vi "Example_CustomCursors.vi"() -> ()   [LabVIEW 2020, in "LcPictureBox.lvclass"]
uses:
  LcPictureBox.lvclass
  SmoothingMode.ctl
  Pen.ctl
  ce328d88-1fef-4cb5-b4df-921596365a82.vi
  1ca8d7fc-782b-495c-9485-1a9aa1dcf8f7.vi
  System.Windows.Forms
panel:
  in  "PictureBox 1":refnum<k24>(container)
  out "error out":errorcluster
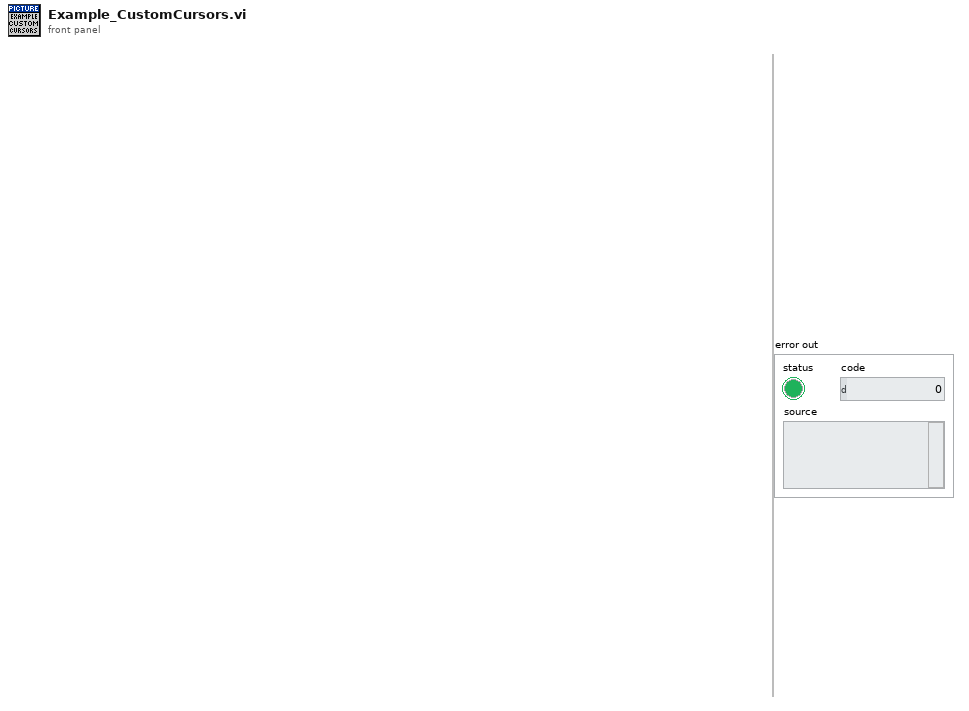
[diagram p1: front panel]
types:
  T1 = typedef "LcPictureBox.lvclass/Pen.ctl" = cluster{"Width":u16, "Style":enum32{"Solid", "Dash", "Dot", "DashDot", "DashDotDot"}}
  T2 = typedef "LcPictureBox.lvclass/SmoothingMode.ctl" = enum16{"None", "HighSpeed", "HighQuality", "AntiAlias"}
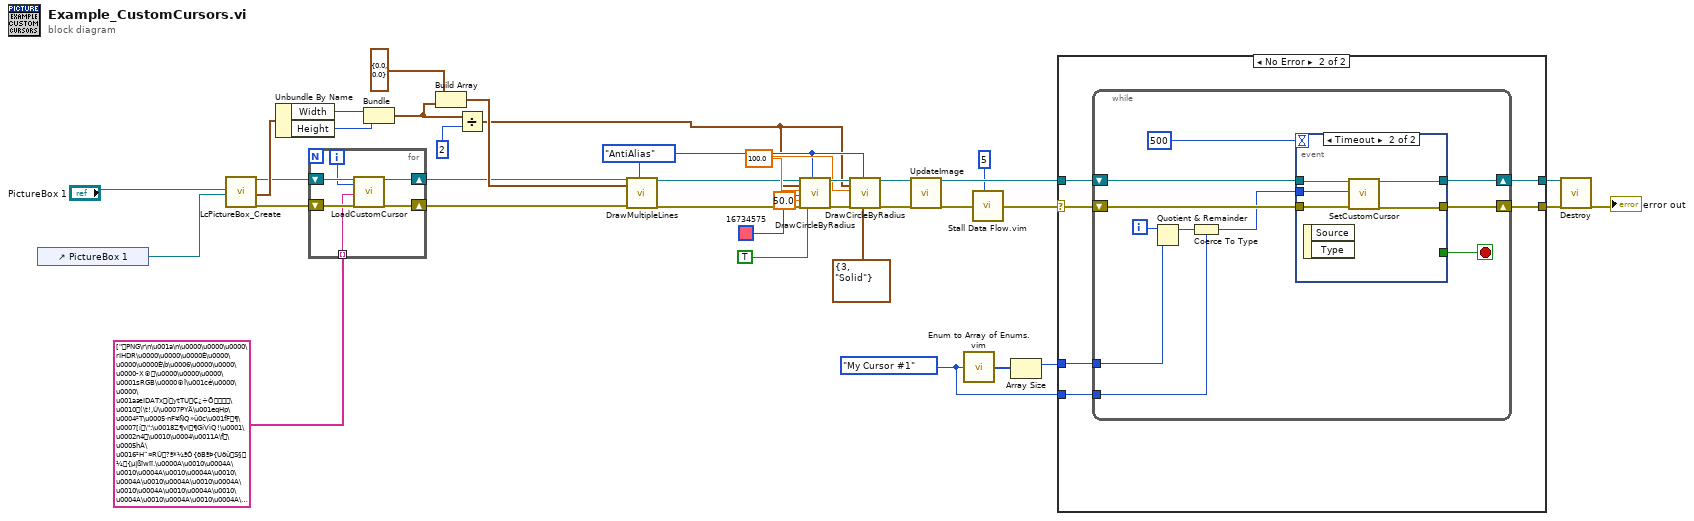
[diagram p0: block diagram]
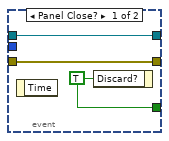
[diagram p3: hidden frame]
diagram:
  w6 = enum16{"My Cursor #1", "My Cursor #2"}."My Cursor #1" ("CursorType")
  w13 = SmoothingMode."AntiAlias" ("SmoothingMode")
  w14 = sgl 100.0 ("Radius")
  n1 = control-ref of="PictureBox 1"() -> (w8:refnum<vi>)
  n2 = call "LcPictureBox_Create.vi"("PictureBox"="PictureBox 1", "PictureBoxActiveXReference"=w8) -> ("reference out"=w4:refnum<class "LcPictureBox.lvclass">, "ImageSizeUsed"=w37:cluster{"Width":i32, "Height":i32}, "Error Out"=w28:errorcluster)  [unwired: 15 in]
  n3 = Unbundle By Name(w37) -> ("Width"=w32:i32, "Height"=w31:i32)
  n4 = for {
    shift-right: [w42] -> w5
    shift-left: w28 -> [w43]
    shift-right: [w40] -> w3
    shift-left: w4 -> [w41]
    tunnel: string[] ["PNG\r\n\u001a\n\u0000\u0000\u0000\rIHDR\u0000\u0000\u0000È\u0000\u0000\u0000È\b\u0006\u0000\u0000\u0000­X®\u0000\u0000\u0000\u0001sRGB\u0000®Î\u001cé\u0000\u0000\u001aæIDATxíytTUÇ¿÷Õ\u0010(\t!,Ú\u0007PYÄ\u001eqHp\u0004²T\u0005·nF¥ÑQ»û0c\u001fF¶\u0007[í\":\u0018Z¶vi¶GíVìQ!\u0001\u0002n4\u0010\u0004\u0011A\f\u0005hÂ\u0016²H¨¤RÛ?ª*¼ªÔ{õBªÞ{UõûS§¼{µ|ßïwïï.\u0000A\u0010\u0004A\u0010\u0004A\u0010\u0004A\u0010\u0004A\u0010\u0004A\u0010\u0004A\u0010\u0004A\u0010\u0004A\u0010\u0004A\u0010\u0004A\u0010\u0004A\u0010\u0004A\u0010\u0004A\u0010\u0004A\u0010\u0004A\u0010\u0004A\u0010\u0004A\u0010\u0004A\u0010\u0004A\u0010\u0004A\u00101\bSÛXÅl6ß\f`\u0016\"ÆØdá5ç\u000f2Æ*ÜnweEEÅçêXHÈ\u0004\u0012Fn½õÖÔÄÄÄ\u0003x\u0004À2ÿí\u001cµz½~í\u001f~Ø\u00129ëË\u0004\u0012&,\u0016Ëb\u0000\u0002H¾ÿçy¾\u0013ÀÊòòò'Âj\u0018Ñ/H ý$???yàÀë\u0001\u0014£>ç?á8î\r\u001b6t£>¢@úÁìÙ³ÓFã'\u0000&¹êoívûÊÊÊÖ0×Kô\u0011Nm\u0003¢üü|½Á`Øð\u0003\u0000®5\u0018\fæçç'D n¢\u000fèÕ6 \na\u0000Xrrr\u0019clTÁ+®¸\u00028q\"233ár¹pæÌ\u0019ìÞ½\u001bhkk\u0013o±ë×\u0001¸\u0017\u0000ï}\u0010\nC!Vß`\u0000XAAÁd½^_Ã\u0018\u000búþét:ÜsÏ=¸ë®» R\u0004v»\u001do¾ù&6mÚ$Ù Ûí6WTTl\u0006D\u0015tj\u001b\u0010ep\u0000¸k®¹f\u000bcì`\u0005ðÌ3Ï //OT\u001cGDS¦LAv...", "PNG\r\n\u001a\n\u0000\u0000\u0000\rIHDR\u0000\u0000\u0000È\u0000\u0000\u0000È\b\u0006\u0000\u0000\u0000­X®\u0000\u0000\u0000\u0001sRGB\u0000®Î\u001cé\u0000\u0000 \u0000IDATxí{x\u0014Uÿ¿UÕÝ¹tî$Üù%`\b÷\u0011PºD\u00194W`UV\u0011\u0011\\qfYwpö÷<?ÝÙq\u001cuwÕY\u001d]W\u001cÀ\u000bà\u000e\u0000ñ\u0002\t \u00100\u0004È\u0005@$$MÒNwªë÷GwuN®êî¤/\tx>ÏÓO:UÕUo]¾õsÞ÷\u00030\u0018\f\u0006Á`0\u0018\f\u0006Á`0\u0018\f\u0006Á`0\u0018\f\u0006Á`0\u0018\f\u0006Á`0\u0018\f\u0006Á`0\u0018\f\u0006Á¸ùáÚ\u0000\u0006PPPp¯ÃáHã8.M¤\u0006INîÞ½ûÄPÛÅ`\u0002\u0019R\n\n\n\u0001x\r@Êê\u0006\u0000ÏîÜ¹sGx­b\bCmÀ÷×\u0000¼\u000e Ac\u0004\u0000L2%¡¦¦æóðYÆ a\u001ed\bpy¿ÒË%I\u0002Ç©Þ¿edh`\u0002\t/\\^^^\u0002Ïóçáò\u001cZ¢ w:\u001cI»víê\u0004 ÍZ\u0006ø¡6à{\u0004çú<\u000b\u001fâ\u0000\u0000ã In-$¸~'ï\u0011&ØÅ\u000e\u000f\u001c\u0000nÑ¢E\u0013FãQh×;¼Ñi±XÒ÷îÝÛ\u0001§\u0017a$\f0\u000f\u0012\u001e8\u0000|ttô¯áE\u001cK,ABæê¨¨¨×à¼gìÅ\u0016&@B\u000f\u0007?þ$ãVim\u0014\u001d\u001d\u0015+Và¡\u001eÒÞ\u0011Ç­?þ$°¢VØ`\u0002\t-òÌÇÇÇÿÊÛË/ÑhDvv6F\u001c©¹k?²\u0017a\"\t1L ¡_¼xñBç\u001fÓÚ >>\u001e\u0005\u0005\u0005\u0000\u0000Á\u0015+Vhïç\u001f[´hÑ\u001c°{\u0017\u0016ØE\u000e\u001d..."] -> [w38] mode=indexing
    i -> [w39]
    n5 = call "LoadCustomCursor.vi"("reference in"=w41, "CustomCusorIndex"=w39, "ImageFileContent"=w38, "error in (no error)"=w43) -> ("reference out"=w40:refnum<class "LcPictureBox.lvclass">, "error out"=w42:errorcluster)  [unwired: 14 in]
  }
  n6 = Bundle("Width"=w32, "Height"=w31) -> (w24:cluster{"Width":i32, "Height":i32})  [unwired: 1 in]
  n7 = Build Array(cluster{"x":dbl, "y":dbl} {"x"=0.0, "y"=0.0} ("Point"), w24) -> (w29:cluster{"x":dbl, "y":dbl}[])
  n8 = Divide(x=w24, y=2) -> (x/y=w10:cluster{"Width":dbl, "Height":dbl})
  n9 = call-dynamic "DrawMultipleLines.vi"("reference in"=w3, "LineEndPoints"=w29, "Error In"=w5, "SmoothingMode(AntiAlias)"=w13) -> ("reference out"=w11:refnum<class "LcPictureBox.lvclass">, "Error Out"=w12:errorcluster)  [unwired: 14 in]
  n10 = call-dynamic "DrawCircleByRadius.vi"("reference in"=w11, "Center"=w10, "Radius"=w14, "Color(Black)"=u32 16734575, "Alpha(100%)"=50.0, "Error In"=w12, "Fill(False)"=TRUE, "SmoothingMode(AntiAlias)"=w13) -> ("reference out"=w18:refnum<class "LcPictureBox.lvclass">, "Error Out"=w16:errorcluster)  [unwired: 10 in]
  n11 = call-dynamic "DrawCircleByRadius.vi"("reference in"=w18, "Center"=w10, "Radius"=w14, "Error In"=w16, "SmoothingMode(AntiAlias)"=w13, "Pen(Width=1, Solid)"=T1 {"Width"=3, "Style"=enum."Solid"}) -> ("reference out"=w17:refnum<class "LcPictureBox.lvclass">, "Error Out"=w15:errorcluster)  [unwired: 12 in]
  n12 = call-dynamic "UpdateImage.vi"("reference in"=w17, "Error In"=w15) -> ("reference out"=w26:refnum<class "LcPictureBox.lvclass">, "Error Out"=w23:errorcluster)  [unwired: 14 in, 2 out]
  n13 = call "Enum to Array of Enums.vim"("enum"=w6) -> ("array of enums"=w2:enum16{"My Cursor #1", "My Cursor #2"}[])
  n14 = call "Stall Data Flow.vim"("value in"=w23, "milliseconds to wait"=u32 5 ("msToWait")) -> ("value out"=w25:errorcluster)  [unwired: 1 out]
  n15 = Array Size(array=w2) -> (size(s)=w7:i32)
  n16 = case shown="No Error" w25 {
    selector: w25 -> [w45 w48]
    tunnel: [w45 w51] -> w35
    tunnel: w26 -> [w44 w50]
    tunnel: [w44 w49] -> w34
    tunnel: w7 -> [_ w47]
    tunnel: w6 -> [_ w46]
    frame Error {
    }
    frame No Error {
      n17 = while {
        shift-right: [w60] -> w49
        shift-left: w50 -> [w61]
        shift-right: [w62] -> w51
        shift-left: w48 -> [w59]
        tunnel: w47 -> [w56]
        tunnel: w46 -> [w54]
        i -> [w53]
        stop <- w58 stop-if-true
        n18 = Quotient & Remainder(x=w53, y=w56) -> (x-y*floor(x/y)=w55:i32)  [unwired: 1 out]
        n19 = Coerce To Type(0:w55, 1:w54) -> (2:w52:enum16{"My Cursor #1", "My Cursor #2"})
        n20 = event shown="[1] Timeout" {
          selector: _ -> [_ _]
          dyn-events: _ -> [_ _]
          timeout: 500 -> [_ _]
          tunnel: w59 -> [w65 w69]
          tunnel: [w65 w68] -> w62
          tunnel: w61 -> [w64 w70]
          tunnel: [w64 w67] -> w60
          tunnel: [w63 _] -> w58
          tunnel: w52 -> [_ w66]
          event Panel Close? {
            w63 = TRUE ("Discard?")
            n21 = event-data() -> ()  [unwired: 1 in, 1 out]
            n22 = event-data("Discard?"=w63) -> ()  [unwired: 1 in, 1 out]
          }
          event Timeout {
            n23 = event-data() -> ()  [unwired: 1 in, 2 out]
            n24 = call-dynamic "SetCustomCursor.vi"("reference in"=w70, "CustomCusorIndex"=w66, "error in (no error)"=w69) -> ("reference out"=w67:refnum<class "LcPictureBox.lvclass">, "error out"=w68:errorcluster)  [unwired: 15 in]
          }
        }
      }
    }
  }
  n25 = call-dynamic "Destroy.vi"("reference in"=w34, "Error In"=w35) -> ("Error Out"=→"error out":errorcluster)  [unwired: 16 in, 1 out]
